vi "RTS Door CMD.vi"(7 "Station":u16=1 min=1 max=8 step=1, 8 "Error In":errorcluster, 9 "Freezer":T1, 10 "Cab":T1, 11 "Slide":T1) -> (0 "Error Out":errorcluster, 3 "Door CMD":string)   [LabVIEW 2020]
uses:
  Drivers/WAGO 750-881/Type Definitions/Wago Door Operation.ctl
  Type Definitions/RTS Custom Commands.ctl
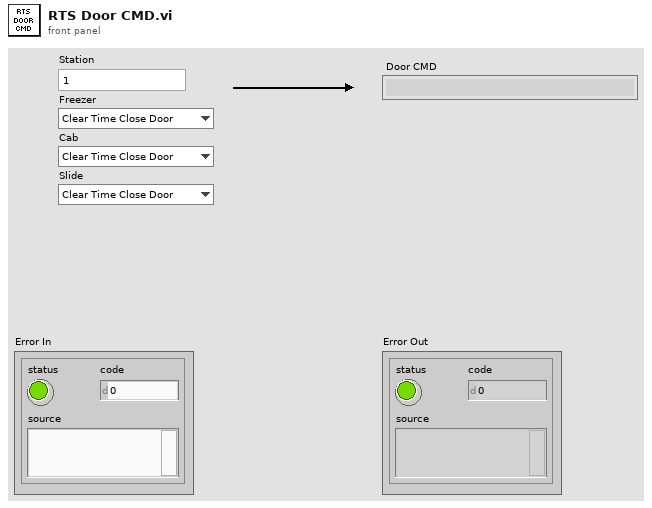
[diagram p1: front panel]
types:
  T1 = typedef "Wago Door Operation.ctl" = enum16{"Clear Time Close Door", "Open Door", "Close Door", "PLC Timed Door Op"}
  T2 = typedef "RTS Custom Commands.ctl" = string
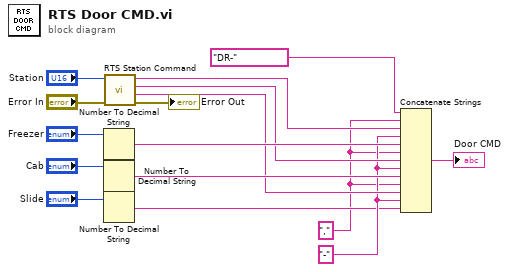
[diagram p0: block diagram]
diagram:
  w5 = "-" ("string")
  w2 = "," ("string")
  n1 = Number To Decimal String(number="Freezer") -> (decimal integer string=w9:string)  [unwired: 1 in]
  n2 = Number To Decimal String(number="Cab") -> (decimal integer string=w7:string)  [unwired: 1 in]
  n3 = Number To Decimal String(number="Slide") -> (decimal integer string=w4:string)  [unwired: 1 in]
  n4 = call "RTS Station Command.vi"("Error In"="Error In", "Station"="Station") -> ("Error Out"=→"Error Out":errorcluster, "Slide"=w6:string, "Cab"=w8:string, "Freezer"=w3:string)  [unwired: 6 in]
  n5 = Concatenate Strings(T2 "DR-" ("string"), w2, w3, w5, w9, w2, w8, w5, w7, w2, w6, w5, w4) -> (→"Door CMD":string)
